vi "Get PXI Device List.vi"(7 "Filter Type":T1=enum."Product Name", 8 "error in (no error)":errorcluster, 10 "Filter Names":string[](array[string]), 11 "Target IP Address":string="10.1.128.170") -> (0 "error out":errorcluster, 2 "Alias":string[](array[string]), 3 "Name and Alias":string[](array[string]))   [LabVIEW 2020, in "NIVS Hardware Discovery.lvlib"]
uses:
  NIVS Hardware Discovery.lvlib
  <vilib>/nisyscfg/nisyscfg.lvlib
  <resource>/objmgr/nicriosae.rc
  _Types/Filter Type.ctl
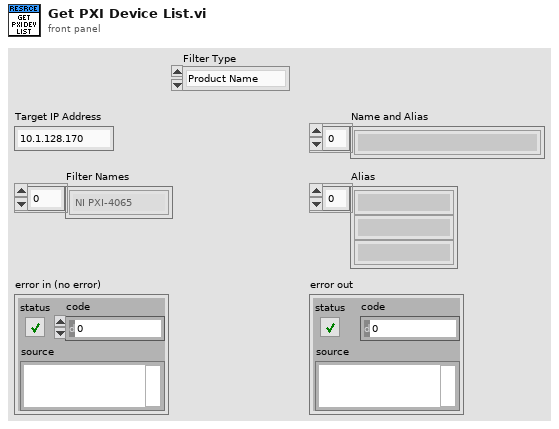
[diagram p1: front panel]
types:
  T1 = typedef "NIVS Hardware Discovery.lvlib/Filter Type.ctl" = enum16{"Device Category", "Product Name", "Ethernet", "XNET", "VISA", "FPGA", "EtherCAT Master", "DAQmx", "GPIB", "Serial"}
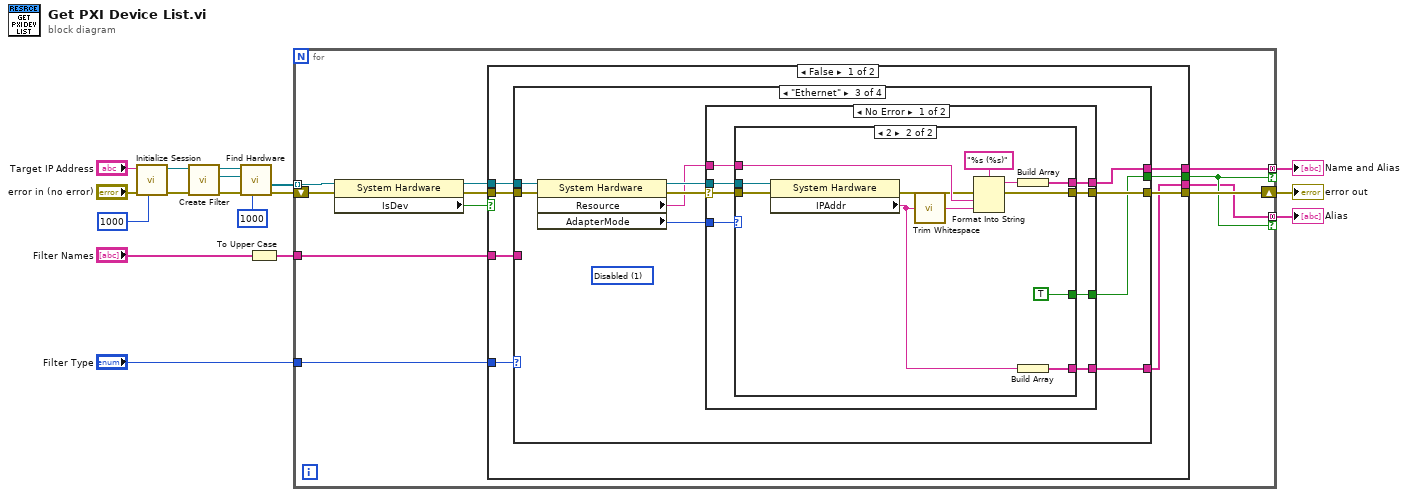
[diagram p0: block diagram]
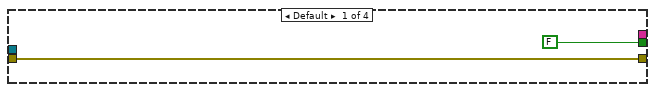
[diagram p2: hidden frame]
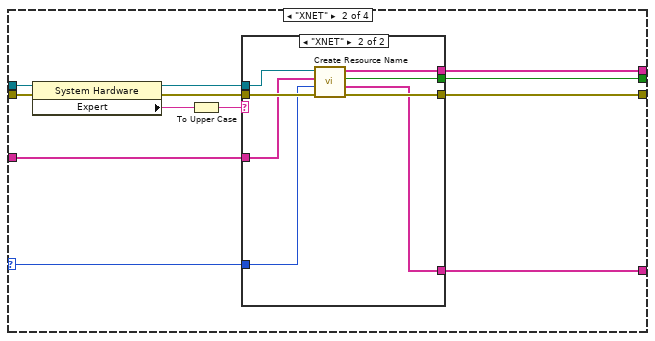
[diagram p3: hidden frame]
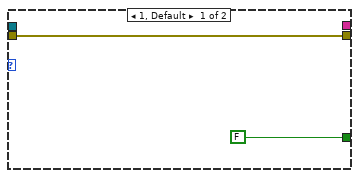
[diagram p5: hidden frame]
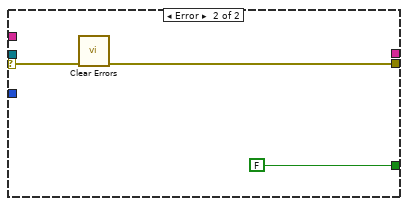
[diagram p6: hidden frame]
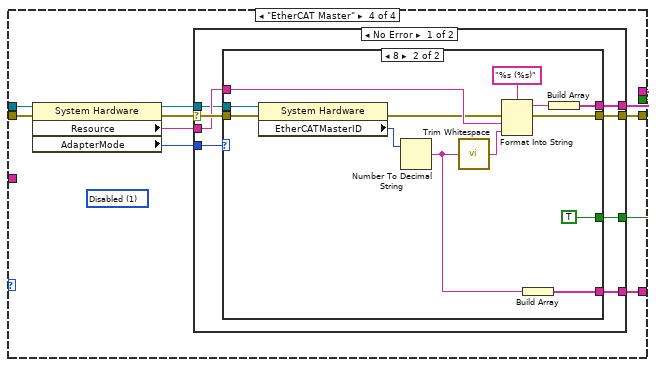
[diagram p7: hidden frame]
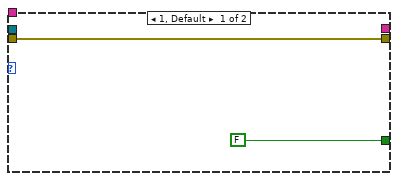
[diagram p8: hidden frame]
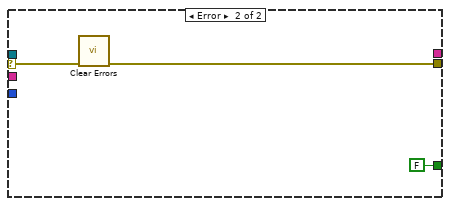
[diagram p9: hidden frame]
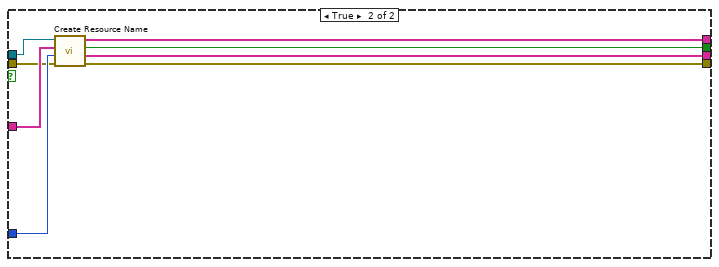
[diagram p10: hidden frame]
diagram:
  n1 = call <vilib>:"Initialize Session.vi"("Connect Timeout (4000 ms)"=u32 1000, "error in (no error)"="error in (no error)", "Target (localhost)"="Target IP Address") -> ("error out"=w9:errorcluster, "Session out"=w7:refnum<k21>)  [unwired: 7 in]
  n2 = call <vilib>:"Create Filter.vi"("error in (no error)"=w9, "Session in"=w7) -> ("error out"=w2:errorcluster, "Filter out"=w1:refnum<k20>, "Session out"=w8:refnum<k21>)  [unwired: 7 in]
  n3 = call <vilib>:"Find Hardware.vi"("Remote Timeout (300,000 ms)"=u32 1000, "error in (no error)"=w2, "Filter in"=w1, "Session in"=w8) -> ("error out"=w11:errorcluster, "Resources out"=w10:refnum<k20>[])  [unwired: 4 in, 2 out]
  n4 = To Upper Case(1:"Filter Names") -> (0:w5:string[])
  n5 = for {
    tunnel: w10 -> [w20] mode=indexing
    tunnel: [w28] -> w13 mode=concatenating if=w25
    shift-right: [w27] -> w14
    shift-left: w11 -> [w22]
    tunnel: [w24] -> w15 mode=concatenating if=w25
    tunnel: w5 -> [w26]
    tunnel: "Filter Type" -> [w23]
    n6 = property class="System Hardware"(reference=w20, error in=w22) -> (reference out=w19:refnum<k20>, error out=w21:errorcluster, "IsDev"=w18:bool)
    n7 = case shown="False" w18 {
      tunnel: [w30 w138] -> w28
      tunnel: [w33 w137] -> w27
      tunnel: w26 -> [w29 w136]
      tunnel: [w32 w135] -> w25
      tunnel: [w31 w134] -> w24
      tunnel: w23 -> [w34 w133]
      tunnel: w21 -> [w36 w132]
      tunnel: w19 -> [w35 w131]
      frame False {
        n8 = case shown="\"Ethernet\"" w34 {
          selector: w34 -> [_ w41 _ _]
          tunnel: w36 -> [w38 w49 w69 w104]
          tunnel: w35 -> [_ w50 w68 w103]
          tunnel: [w38 w45 w65 w100] -> w33
          tunnel: [FALSE w44 w64 w99] -> w32
          tunnel: [_ w39 w62 w97] -> w31
          tunnel: [_ w40 w61 w96] -> w30
          tunnel: w29 -> [_ w42 _ _]
          frame Default {
          }
          frame "XNET" {
            n9 = property class="System Hardware"(reference=w50, error in=w49) -> (reference out=w46:refnum<k20>, error out=w47:errorcluster, "Expert"=w48:string)
            n10 = To Upper Case(1:w48) -> (0:w43:string)
            n11 = case shown="\"XNET\"" w43 {
              tunnel: w47 -> [w51 w59]
              tunnel: w46 -> [_ w57]
              tunnel: [w51 w58] -> w45
              tunnel: [_ w52] -> w44
              tunnel: w42 -> [_ w56]
              tunnel: w41 -> [_ w55]
              tunnel: [_ w54] -> w40
              tunnel: [_ w53] -> w39
              frame Default {
              }
              frame "XNET" {
                n12 = call "Create Resource Name.vi"("error in (no error)"=w59, "Filter Type"=w55, "Filter List"=w56, "System Hardware Ref"=w57) -> ("error out"=w58:errorcluster, "Alias"=w53:string[], "Use"=w52:bool, "Name and Alias"=w54:string[])  [unwired: 4 in]
              }
            }
          }
          frame "Ethernet" {
            (unwired) u32 1 items=["Disabled"=1, "TCP/IP Ethernet"=2, "Deterministic"=4, "EtherCAT"=8, "TCP/IP WLAN Connect"=32, "TCP/IP WLAN Create"=64] ("Network Adapters:Adapter Mode")
            n13 = property class="System Hardware"(reference=w68, error in=w69) -> (reference out=w63:refnum<k20>, error out=w66:errorcluster, "Resource"=w60:string, "AdapterMode"=w67:u32)
            n14 = case shown="No Error" w66 {
              selector: w66 -> [w76 w94]
              tunnel: w67 -> [w77 _]
              tunnel: [w71 w93] -> w65
              tunnel: w60 -> [w75 _]
              tunnel: [w74 FALSE] -> w64
              tunnel: w63 -> [w73 _]
              tunnel: [w72 _] -> w62
              tunnel: [w70 _] -> w61
              frame No Error {
                n15 = case shown="2" w77 {
                  tunnel: w76 -> [w78 w89]
                  tunnel: w75 -> [_ w87]
                  tunnel: [FALSE TRUE] -> w74
                  tunnel: w73 -> [_ w88]
                  tunnel: [_ w80] -> w72
                  tunnel: [w78 w84] -> w71
                  tunnel: [_ w81] -> w70
                  frame 1, Default {
                  }
                  frame 2 {
                    n16 = property class="System Hardware"(reference=w88, error in=w89) -> (error out=w85:errorcluster, "IPAddr"=w86:string)  [unwired: 1 out]
                    n17 = call-poly <vilib>:"Trim Whitespace.vi"("string"=w86) -> ("trimmed string"=w91:string)  [unwired: 1 in]
                    n18 = Format Into String(format string="%s (%s)", error in=w85, w87, w91) -> (resulting string=w82:string, error out=w84:errorcluster)  [unwired: 1 in]
                    n19 = Build Array(w82) -> (w81:string[])
                    n20 = Build Array(w86) -> (w80:string[])
                  }
                }
              }
              frame Error {
                n21 = call <vilib>:"Clear Errors.vi"("error in (no error)"=w94) -> ("error out"=w93:errorcluster)  [unwired: 5 in, 1 out]
              }
            }
          }
          frame "EtherCAT Master" {
            (unwired) u32 1 items=["Disabled"=1, "TCP/IP Ethernet"=2, "Deterministic"=4, "EtherCAT"=8, "TCP/IP WLAN Connect"=32, "TCP/IP WLAN Create"=64] ("Network Adapters:Adapter Mode")
            n22 = property class="System Hardware"(reference=w103, error in=w104) -> (reference out=w98:refnum<k20>, error out=w101:errorcluster, "Resource"=w95:string, "AdapterMode"=w102:u32)
            n23 = case shown="No Error" w101 {
              selector: w101 -> [w111 w130]
              tunnel: w102 -> [w112 _]
              tunnel: [w106 w129] -> w100
              tunnel: w95 -> [w110 _]
              tunnel: [w109 FALSE] -> w99
              tunnel: w98 -> [w108 _]
              tunnel: [w107 _] -> w97
              tunnel: [w105 _] -> w96
              frame No Error {
                n24 = case shown="8" w112 {
                  tunnel: w111 -> [w113 w125]
                  tunnel: w110 -> [_ w123]
                  tunnel: [FALSE TRUE] -> w109
                  tunnel: w108 -> [_ w124]
                  tunnel: [_ w117] -> w107
                  tunnel: [w113 w121] -> w106
                  tunnel: [_ w118] -> w105
                  frame 1, Default {
                  }
                  frame 8 {
                    n25 = property class="System Hardware"(reference=w124, error in=w125) -> (error out=w122:errorcluster, "EtherCATMasterID"=w116:u32)  [unwired: 1 out]
                    n26 = Number To Decimal String(number=w116) -> (decimal integer string=w115:string)  [unwired: 1 in]
                    n27 = call-poly <vilib>:"Trim Whitespace.vi"("string"=w115) -> ("trimmed string"=w127:string)  [unwired: 1 in]
                    n28 = Format Into String(format string="%s (%s)", error in=w122, w123, w127) -> (resulting string=w119:string, error out=w121:errorcluster)  [unwired: 1 in]
                    n29 = Build Array(w115) -> (w117:string[])
                    n30 = Build Array(w119) -> (w118:string[])
                  }
                }
              }
              frame Error {
                n31 = call <vilib>:"Clear Errors.vi"("error in (no error)"=w130) -> ("error out"=w129:errorcluster)  [unwired: 5 in, 1 out]
              }
            }
          }
        }
      }
      frame True {
        n32 = call "Create Resource Name.vi"("error in (no error)"=w132, "Filter Type"=w133, "Filter List"=w136, "System Hardware Ref"=w131) -> ("error out"=w137:errorcluster, "Alias"=w134:string[], "Use"=w135:bool, "Name and Alias"=w138:string[])  [unwired: 4 in]
      }
    }
  }
  "Name and Alias" <- w13
  "Alias" <- w15
  "error out" <- w14
